vi "BusB_Acquire.vi"(8 "error in (no error)":errorcluster, 11 "BusB VISA resource in":refnum<visa-resource-name>) -> (0 "error out":errorcluster, 1 "Match & Update":bool, 2 "BusB Raw Data":u8[](array[numeric]), 3 "BusB VISA resource out":refnum<visa-resource-name>)   [LabVIEW 2016, in "Impedance Data Acquisition and Decoding.lvlib"]
uses:
  Impedance Data Acquisition and Decoding.lvlib
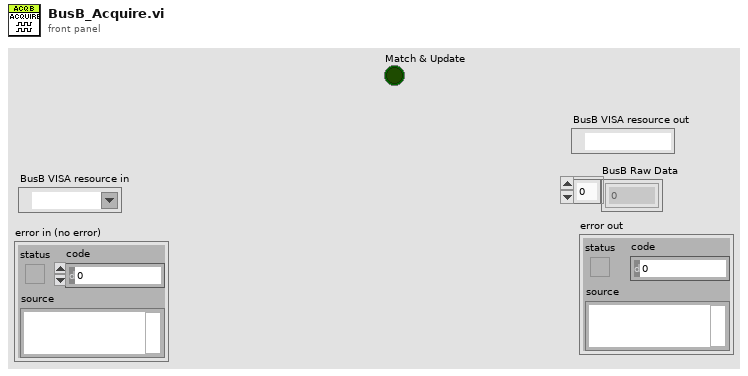
[diagram p1: front panel]
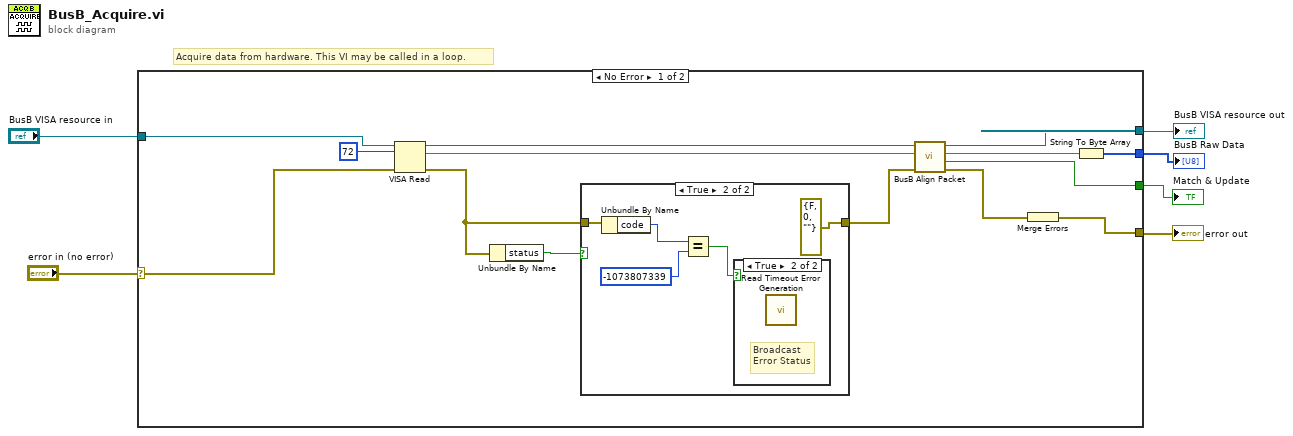
[diagram p0: block diagram]
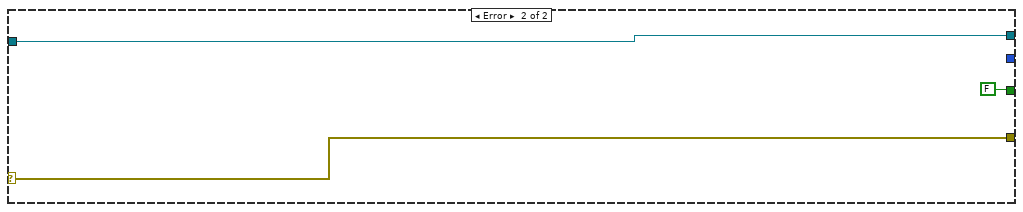
[diagram p4: hidden frame]
diagram:
  # "Acquire data from hardware. This VI may be called in a loop."
  n1 = case shown="No Error" "error in (no error)" {
    selector: "error in (no error)" -> [w16 w29]
    tunnel: [w19 w29] -> w5
    tunnel: "BusB VISA resource in" -> [w17 w28]
    tunnel: [w20 _] -> w3
    tunnel: [w11 w28] -> w2
    tunnel: [w7 FALSE] -> w1
    frame No Error {
      n2 = VISA Read(VISA resource name=w17, byte count=u32 72, error in (no error)=w16) -> (VISA resource name out=w12:refnum<visa-resource-name>, read buffer=w15:string, error out=w9:errorcluster)  [unwired: 1 out]
      n3 = Unbundle By Name(w9) -> ("status"=w10:bool)
      n4 = case shown="True" w10 {
        tunnel: w9 -> [w21 w24]
        tunnel: [w21 errorcluster {"status"=FALSE, "code"=0, "source"=""} ("error constant")] -> w8
        frame False {
        }
        frame True {
          n5 = Unbundle By Name(w24) -> ("code"=w26:i32)
          n6 = Equal?(x=w26, y=-1073807339 ("code")) -> (x = y?=w22:bool)
          n7 = case shown="True" w22 {
            frame False {
            }
            frame True {
              # "Broadcast\nError Status"
              n8 = call "Read Timeout Error Generation.vi"() -> ()  [unwired: 11 in, 1 out]
            }
          }
        }
      }
      n9 = call "BusB Align Packet.vi"("error in"=w8, "String In"=w15, "VISA resource in"=w12) -> ("error out"=w14:errorcluster, "Match & Update"=w7:bool, "String Out"=w13:string, "VISA resource out"=w11:refnum<visa-resource-name>)  [unwired: 5 in]
      n10 = Merge Errors(w14) -> (w19:errorcluster)
      n11 = String To Byte Array(string=w13) -> (unsigned byte array=w20:u8[])
    }
    frame Error {
    }
  }
  "error out" <- w5
  "BusB Raw Data" <- w3
  "BusB VISA resource out" <- w2
  "Match & Update" <- w1
